vi "Fast Hilbert Transform PtByPt.vi"(2 "initialize":bool, 3 "sample length":i32=100, 5 "x":dbl format="%0.2f") -> (0 "error":i32, 1 "Hilbert{X}":dbl[](array[numeric]))   [LabVIEW 2017, in "NI_PtbyPt.lvlib"]
doc: "Computes the fast Hilbert transform of the set of input data points specified by <B>sample length</B> using fast Fourier transform (FFT) identities."
uses:
  <vilib>/ptbypt/NI_PtbyPt.lvlib
  <vilib>/Analysis/2dsp.llb/Inverse Real FFT.vi
  <vilib>/Analysis/NI_AALPro.lvlib
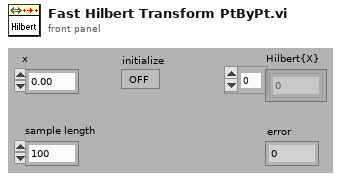
[diagram p1: front panel]
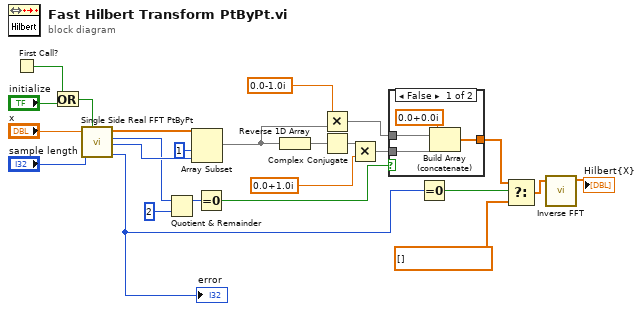
[diagram p0: block diagram]
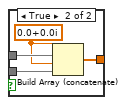
[diagram p2: hidden frame]
diagram:
  n1 = First Call?() -> (First Call?: T/F=w1:bool)
  n2 = Or(x=w1, y="initialize") -> (x .or. y?=w2:bool)
  n3 = call <vilib>:"Single Side Real FFT PtByPt.vi"("initialize"=w2, "sample length"="sample length", "input data"="x") -> ("error"=w3:i32, "half length"=w16:i32, "sample length"=w11:i32, "FFT Single Side"=w12:cdb[])  [unwired: 2 in]
  "error" <- w3
  n4 = Quotient & Remainder(x=w11, y=2) -> (x-y*floor(x/y)=w9:i32)  [unwired: 1 out]
  n5 = Array Subset(array=w12, index=1 ("Array Index"), length=w16) -> (w23:cdb[])
  n6 = Equal To 0?(x=w9) -> (x = 0?=w8:bool)
  n7 = Reverse 1D Array(array=w23) -> (reversed array=w24:cdb[])
  n8 = Multiply(x=cdb 0.0-1.0i, y=w23) -> (x*y=w19:cdb[])
  n9 = Complex Conjugate(1:w24) -> (0:w21:cdb[])
  n10 = Multiply(x=w21, y=cdb 0.0+1.0i) -> (x*y=w18:cdb[])
  n11 = case shown="False" w8 {
    tunnel: w19 -> [w29 w33]
    tunnel: w18 -> [w28 w32]
    tunnel: [w26 w31] -> w7
    frame False {
      n12 = Build Array (concatenate)(cdb 0.0+0.0i, w29, w28) -> (w26:cdb[])
    }
    frame True {
      w30 = cdb 0.0+0.0i
      n13 = Build Array (concatenate)(w30, w33, w30, w32) -> (w31:cdb[])
    }
  }
  n14 = Equal To 0?(x=w3) -> (x = 0?=w5:bool)
  n15 = Select(t=w7, s=w5, f=cdb[] []) -> (s? t:f=w6:cdb[])
  n16 = call-poly <vilib>:"Inverse FFT.vi"("FFT {X}"=w6) -> ("X"=→"Hilbert{X}":dbl[])  [unwired: 9 in, 1 out]
